vi "Set Manager.vi"(10 "Manager":refnum<class "WebSocket Manager.lvclass">, 11 "WebSocket Client in":refnum<class "WebSocket Client.lvclass">) -> (3 "WebSocket Client out":refnum<class "WebSocket Client.lvclass">)   [LabVIEW 2020, in "HTTP Server.lvlib" / "WebSocket Client.lvclass"]
uses:
  WebSocket Client.lvclass
  WebSocket Client.lvclass/WebSocket Client.ctl
  WebSocket Manager/WebSocket Manager.lvclass
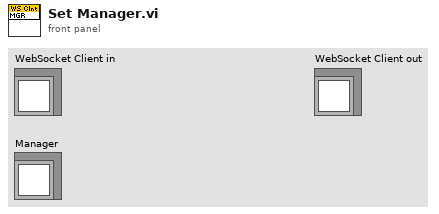
[diagram p1: front panel]
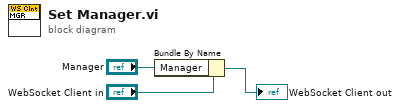
[diagram p0: block diagram]
diagram:
  n1 = Bundle By Name(cluster="WebSocket Client in", "Manager"="Manager") -> (→"WebSocket Client out":refnum<class "WebSocket Client.lvclass">)
